vi "Set Motor Direction.vi"(8 "error in (no error)":errorcluster, 9 "Direction":T1, 10 "Motor":u16, 11 "Motor Controller in":refnum<class "Motor Controller.lvclass">) -> (0 "error out":errorcluster, 3 "Motor Controller out":refnum<class "Motor Controller.lvclass">)   [LabVIEW 2020, in "CTI-Peripheral.lvlib" / "Motor Controller.lvclass"]
uses:
  Motor Controller.lvclass
  Direction.ctl
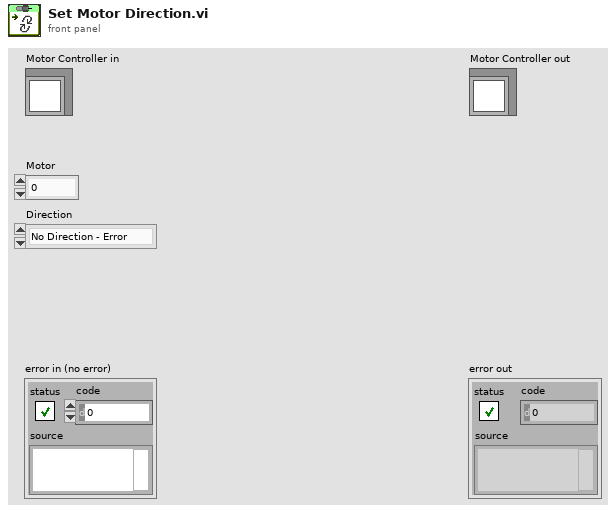
[diagram p1: front panel]
types:
  T1 = typedef "CTI-Peripheral.lvlib/Motor Controller.lvclass/Direction.ctl" = enum16{"No Direction - Error", "Clockwise (CW)", "Anti-Clockwise (ACW)"}
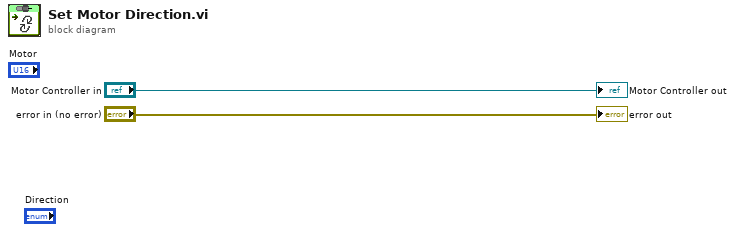
[diagram p0: block diagram]
diagram:
  "error out" <- "error in (no error)"
  "Motor Controller out" <- "Motor Controller in"
